vi "BL_StopChannel.vi"(8 "error in (no error)":errorcluster, 10 "Channel":u8, 11 "Potentiostat Galvanostat in":refnum<class "Potentiostat Galvanostat.lvclass">) -> (0 "error out":errorcluster, 2 "Channel":u8, 3 "Potentiostat Galvanostat out":refnum<class "Potentiostat Galvanostat.lvclass">)   [LabVIEW 2018, in "Potentiostat Galvanostat.lvclass"]
doc: "The hardware conf object. The attribute “Conn” is the electrode\nconnection mode and the attribute “Ground” is the instrument\nground. See 5. Structures and Constants to have the value of these\nattributes."
uses:
  Potentiostat Galvanostat.lvclass
  Potentiostat Galvanostat.lvclass/Potentiostat Galvanostat.ctl
  BL_GetErrorMsg.vi
  <vilib>/Utility/error.llb/Error Cluster From Error Code.vi
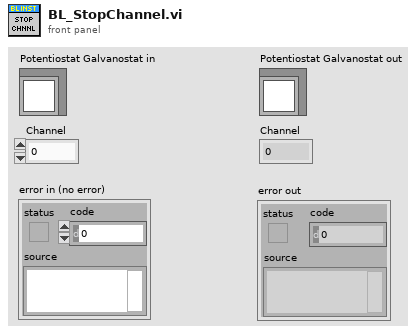
[diagram p1: front panel]
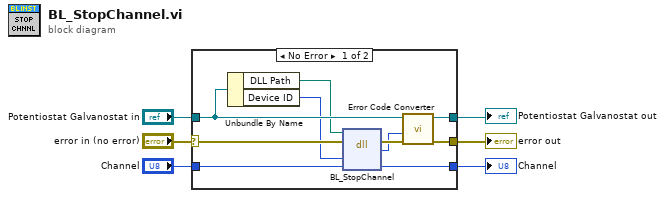
[diagram p0: block diagram]
diagram:
  n1 = case shown="No Error" "error in (no error)" {
    selector: "error in (no error)" -> [w11 w18]
    tunnel: [w16 w18] -> w5
    tunnel: [w15 w17] -> w3
    tunnel: "Potentiostat Galvanostat in" -> [w14 w17]
    tunnel: "Channel" -> [w9 _]
    tunnel: [w8 _] -> w1
    frame No Error {
      n2 = Unbundle By Name(w14) -> ("DLL Path"=w13:path, "Device ID"=w10:i32)
      n3 = dll-call lib="C:/Program Files (x86)/National Instruments/LabVIEW 2018/user.lib/EClib/EClib.*" fn="BL_StopChannel"(path in=w13, error in=w11, "Device ID"=w10, "Channel"=w9) -> (error out=w12:errorcluster, "Error Code"=w7:i32, "Channel"=w8:u8)  [unwired: 2 in, 1 out]
      n4 = call "Error Code Converter.vi"("error in (no error)"=w12, "Error Code"=w7, "Potentiostat Galvanostat in"=w14) -> ("error out"=w16:errorcluster, "Potentiostat Galvanostat out"=w15:refnum<class "Potentiostat Galvanostat.lvclass">)  [unwired: 7 in]
    }
    frame Error {
    }
  }
  "error out" <- w5
  "Potentiostat Galvanostat out" <- w3
  "Channel" <- w1
